vi "Parameter state to short.vi"(10 "STATE":T2) -> (2 "STATE short":T1)   [LabVIEW 2019, in "Inputs.lvlib"]
uses:
  Inputs.lvlib
  Parameter State.ctl
  Parameter State short.ctl
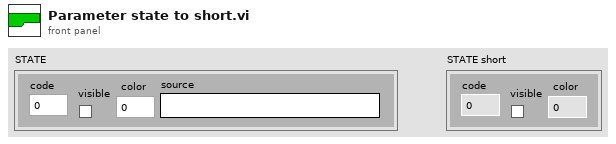
[diagram p1: front panel]
types:
  T1 = typedef "Inputs.lvlib/Parameter State short.ctl" = cluster{"code":i32, "visible":bool, "color":u32}
  T2 = typedef "Inputs.lvlib/Parameter State.ctl" = cluster{"code":i32, "visible":bool, "color":u32, "source":string}
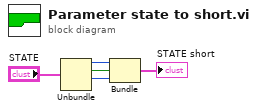
[diagram p0: block diagram]
diagram:
  n1 = Unbundle("STATE") -> ("code"=w4:i32, "visible"=w3:bool, "color"=w2:u32)  [unwired: 1 out]
  n2 = Bundle("code"=w4, "visible"=w3, "color"=w2) -> (→"STATE short":cluster{"code":i32, "visible":bool, "color":u32})  [unwired: 1 in]
